vi "GetPossibleErrorCodes.vi"(8 "error in (no error)":errorcluster caption="Fehler (Eingang, kein Fehler)", 11 "Dictionary Eingang":refnum<class "Dictionary.lvclass"> caption="DNL_LabVIEW Object in") -> (0 "error out":errorcluster caption="Fehler (Ausgang)", 3 "Dictionary Ausgang":refnum<class "Dictionary.lvclass"> caption="DNL_LabVIEW Object out")   [LabVIEW 2013]
uses:
  Dictionary.lvclass
  <vilib>/Utility/error.llb/Error Cluster From Error Code.vi
  <vilib>/ErrorRing/Error Ring.xnode
panel:
  out "Fehler (Ausgang)":errorcluster
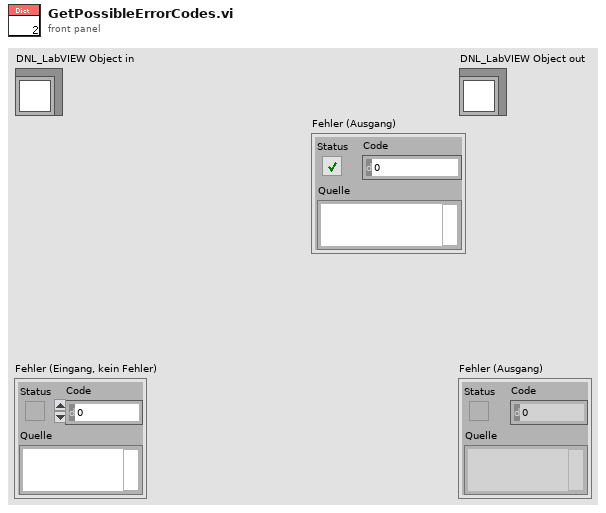
[diagram p1: front panel]
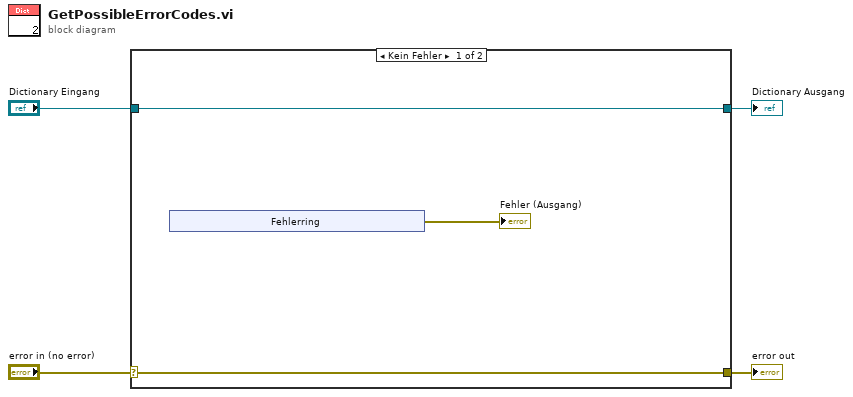
[diagram p0: block diagram]
diagram:
  n1 = case shown="Kein Fehler" "error in (no error)" {
    selector: "error in (no error)" -> [w6 w14]
    tunnel: [w6 w14] -> w3
    tunnel: [w7 w13] -> w1
    tunnel: "Dictionary Eingang" -> [w7 w13]
    frame No Error {
      n2 = xnode "Fehlerring"() -> ("Fehler (Ausgang)"=→"Fehler (Ausgang)":errorcluster)
    }
    frame Error {
    }
  }
  "error out" <- w3
  "Dictionary Ausgang" <- w1
